vi "Wait for axes to stop.vi"(0 "System no.":i32=1, 2 "Axes to wait for":string[](array[string]), 3 "With status bit polling?":bool, 4 "Timeout (s)":dbl=300.0 min=1.0 max=4.0 step=1.0 format="%.2f", 5 "error in":errorcluster, 7 "Polling cycle time, ms":u32=400, 12 "Stop refnum":refnum<vi>) -> (14 "Stopped":bool, 19 "error out":errorcluster)   [LabVIEW 2020]
doc: "This VI waits for the specified axes to stop using #5 polling. It also stops if a communication error occured, Stop refnum or Local stop is TRUE. Requires STA?.vi to be present. Required by General wait for movement to stop.vi. When using as a sub-VI, use Stop refnum to stop VI from caller.\n\nC-880: With status bit polling? = TRUE\n\nAll other systems: With status bit polling? = FALSE"
panel:
  in  "Local stop":bool
  # "This vi waits for the specified axes to stop using #5 polling. \nIt also stops if a communications error occured, Stop refnum\nor Local stop is TRUE."
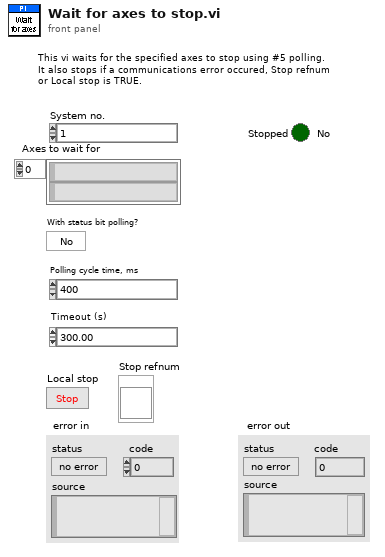
[diagram p1: front panel]
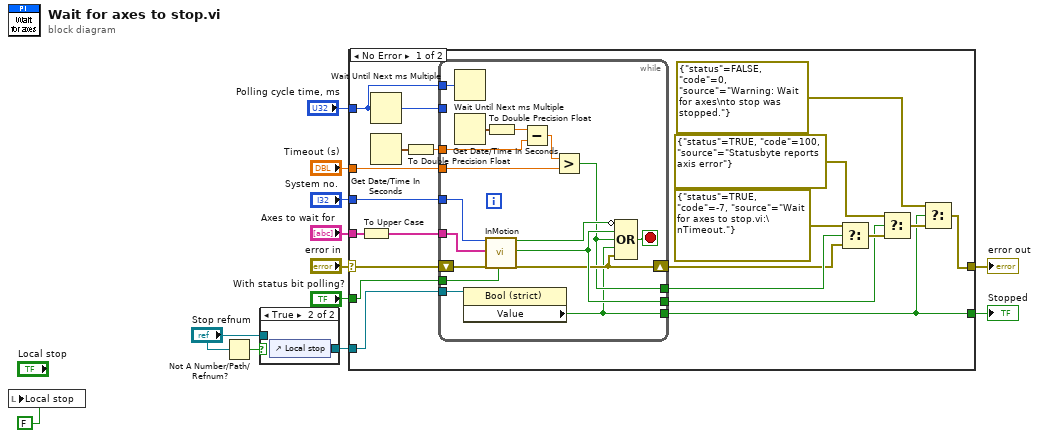
[diagram p0: block diagram]
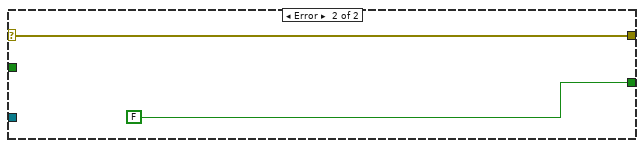
[diagram p3: hidden frame]
diagram:
  n1 = local write "Local stop"(FALSE ("Local stop")) -> ()
  n2 = Not A Number/Path/Refnum?(number/path/refnum="Stop refnum") -> (NaN/Path/Refnum?=w7:bool)
  n3 = case shown="True" w7 {
    tunnel: [w13 w14] -> w6
    tunnel: "Stop refnum" -> [w13 _]
    frame False {
    }
    frame True {
      n4 = control-ref of="Local stop"() -> (w14:refnum<vi>)
    }
  }
  n5 = case shown="No Error" "error in" {
    selector: "error in" -> [w15 w54]
    tunnel: "System no." -> [w35 _]
    tunnel: "Axes to wait for" -> [w29 _]
    tunnel: [w18 w54] -> w12
    tunnel: "With status bit polling?" -> [w33 _]
    tunnel: "Polling cycle time, ms" -> [w17 _]
    tunnel: w6 -> [w34 _]
    tunnel: [w20 FALSE ("Value")] -> w5
    tunnel: "Timeout (s)" -> [w30 _]
    frame No Error {
      n6 = To Upper Case(1:w29) -> (0:w28:string[])
      n7 = Wait Until Next ms Multiple(millisecond multiple=w17) -> (millisecond timer value=w16:u32)
      n8 = Get Date/Time In Seconds() -> (seconds since 1Jan1904=w32:timestamp)
      n9 = To Double Precision Float(number=w32) -> (double precision float=w31:dbl)
      n10 = while {
        tunnel: w28 -> [w43]
        tunnel: w35 -> [w42]
        tunnel: w34 -> [w52]
        tunnel: w33 -> [w38]
        tunnel: [w40] -> w23
        tunnel: w31 -> [w48]
        tunnel: w30 -> [w46]
        tunnel: w17 -> [w45]
        tunnel: [w37] -> w26
        tunnel: [w36] -> w20
        shift-right: [w39] -> w22
        shift-left: w15 -> [w44]
        tunnel: w16 -> [_]
        stop <- w51 stop-if-true
        n11 = Wait Until Next ms Multiple(millisecond multiple=w45) -> ()  [unwired: 1 out]
        n12 = Get Date/Time In Seconds() -> (seconds since 1Jan1904=w50:timestamp)
        n13 = property class="Bool (strict)"(reference=w52) -> ("Value"=w36:bool)  [unwired: 1 in, 2 out]
        n14 = call "InMotion.vi"("System no."=w42, "Axes to check"=w43, "error in (no error)"=w44, "With status bit polling?"=w38) -> ("InMotion"=w41:bool, "Motion Error"=w40:bool, "error out"=w39:errorcluster)  [unwired: 13 in]
        n15 = To Double Precision Float(number=w50) -> (double precision float=w49:dbl)
        n16 = Subtract(x=w49, y=w48) -> (x-y=w47:dbl)
        n17 = Greater?(x=w47, y=w46) -> (0:w37:bool)
        n18 = Compound Arithmetic op=OR(invert w41, w40, w37, w36, w39) -> (w51:bool)
      }
      n19 = Select(t=errorcluster {"status"=TRUE, "code"=-7, "source"="Wait for axes to stop.vi:\nTimeout."} ("error out"), s=w26, f=w22) -> (s? t:f=w25:errorcluster)
      n20 = Select(t=errorcluster {"status"=TRUE, "code"=100, "source"="Statusbyte reports axis error"} ("error out"), s=w23, f=w25) -> (s? t:f=w21:errorcluster)
      n21 = Select(t=errorcluster {"status"=FALSE, "code"=0, "source"="Warning: Wait for axes\nto stop was stopped."} ("error out"), s=w20, f=w21) -> (s? t:f=w18:errorcluster)
    }
    frame Error {
    }
  }
  "error out" <- w12
  "Stopped" <- w5
